vi "Apply SourceInclusion Setting.vi"(7 "Source Index":i32, 8 "error in (no error)":errorcluster, 11 "ProjectItem in":refnum<vi>) -> (0 "error out":errorcluster, 3 "ProjectItem out":refnum<vi>)   [LabVIEW 2019, in "Project Sync Tools.lvclass"]
uses:
  Project Sync Tools.lvclass
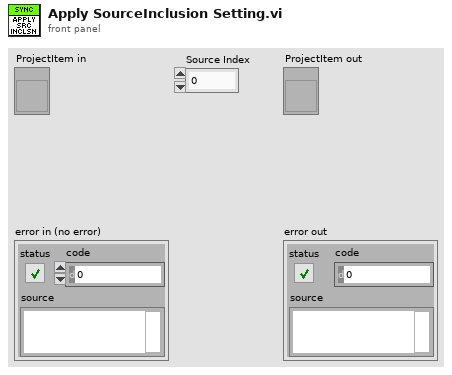
[diagram p1: front panel]
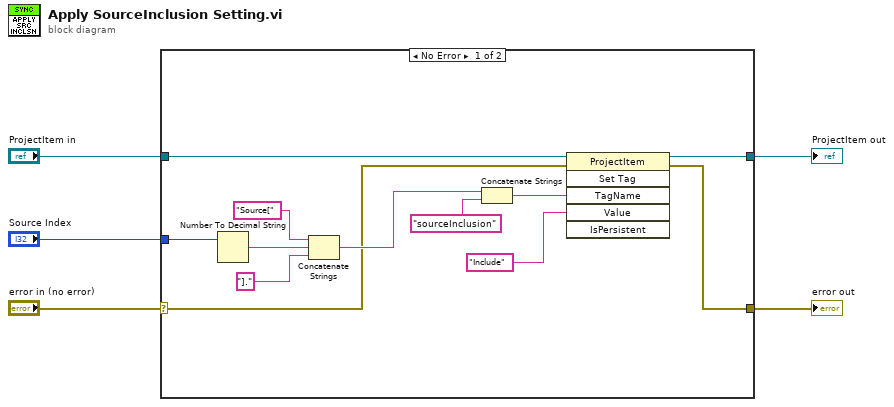
[diagram p0: block diagram]
diagram:
  n1 = case shown="No Error" "error in (no error)" {
    selector: "error in (no error)" -> [w6 w19]
    tunnel: "ProjectItem in" -> [w14 w18]
    tunnel: [w13 w18] -> w4
    tunnel: [w12 w19] -> w3
    tunnel: "Source Index" -> [w8 _]
    frame No Error {
      n2 = Number To Decimal String(number=w8) -> (decimal integer string=w10:string)  [unwired: 1 in]
      n3 = Concatenate Strings("Source[" ("string"), w10, "].") -> (w7:string)
      n4 = Concatenate Strings(w7, "sourceInclusion") -> (w17:string)
      n5 = invoke class="ProjectItem" method="Set Tag"(reference=w14, error in=w6, "TagName"=w17, "Value"="Include") -> (reference out=w13:refnum<vi>, error out=w12:errorcluster)  [unwired: 2 in, 4 out]
    }
    frame Error {
    }
  }
  "ProjectItem out" <- w4
  "error out" <- w3
